vi "Encoder Quad Phase Detection.vi"(8 "Phase B":bool, 9 "Phase A":bool, 10 "Clear Error?":bool, 11 "Enable?":bool) -> (1 "Signal":bool, 2 "Backward?":bool, 3 "Error":bool)   [LabVIEW 2019]
uses:
  Encoder States.ctl
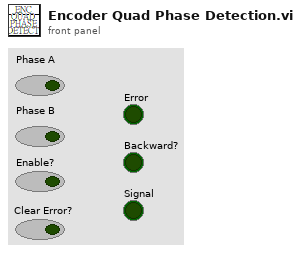
[diagram p1: front panel]
types:
  T1 = typedef "Encoder States.ctl" = fxp<+,3,3>
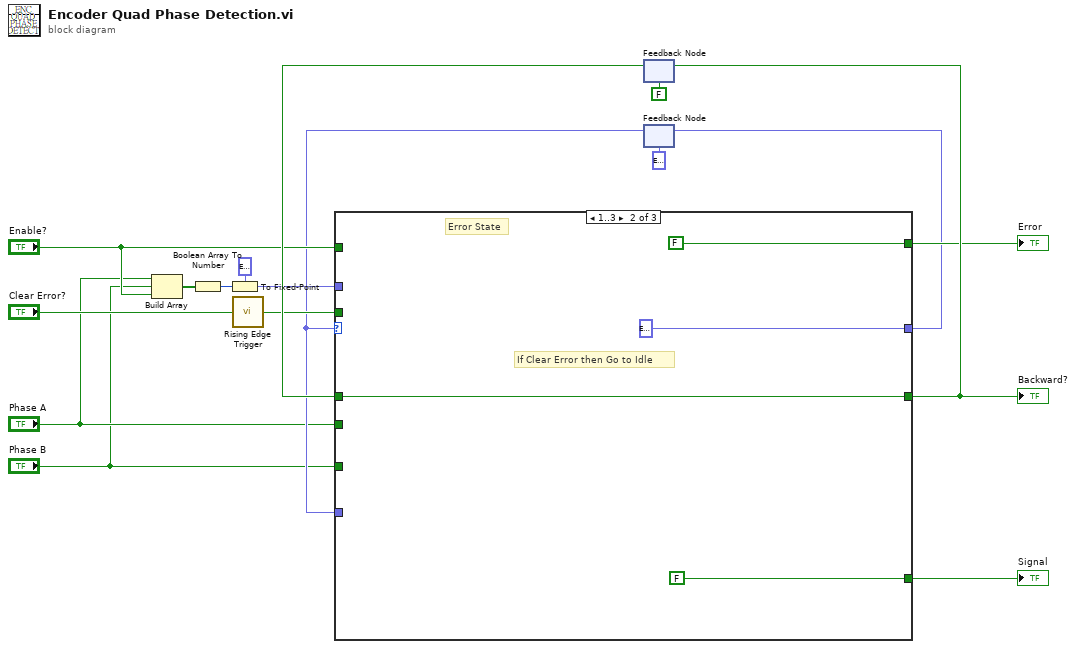
[diagram p0: block diagram]
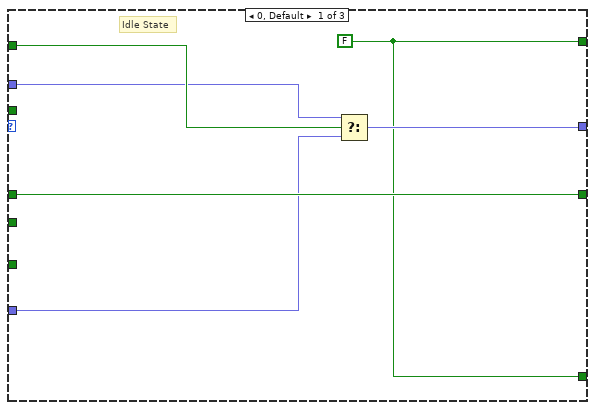
[diagram p2: hidden frame]
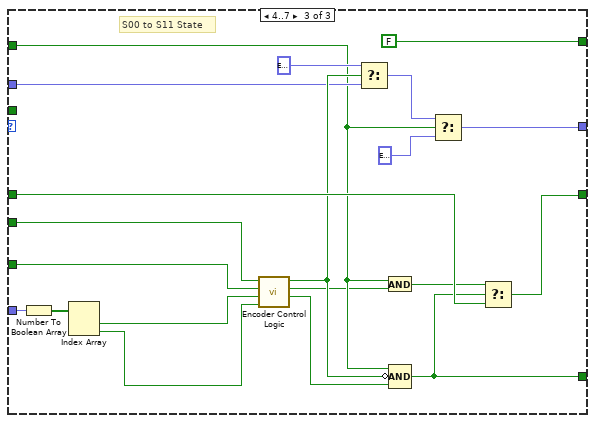
[diagram p3: hidden frame]
diagram:
  n1 = Build Array("Phase A", "Phase B", "Enable?") -> (w6:bool[])
  n2 = Boolean Array To Number(Boolean array=w6) -> (number=w5:u8)
  n3 = To Fixed-Point(fixed-point type=T1 0.0 ("Numeric"), number=w5) -> (fixed-point=w3:T1)
  n4 = call "Rising Edge Trigger.vi"("Signal"="Clear Error?") -> ("Trigger?"=w9:bool)
  n5 = feedback #1(FALSE ("Direction")) -> (w11:bool)
  n6 = feedback #2(T1 0.0) -> (w7:T1)
  n7 = case shown="1..3" w7 {
    tunnel: "Enable?" -> [w23 _ w34]
    tunnel: [w21 T1 0.0 ("t") w38] -> w13
    tunnel: [w19 FALSE ("Error") FALSE ("Error")] -> w15
    tunnel: w3 -> [w22 _ w42]
    tunnel: w11 -> [w20 w26 w47]
    tunnel: [w20 w26 w46] -> w16
    tunnel: [w19 FALSE ("Error") w36] -> w17
    tunnel: w9 -> [_ _ _]
    tunnel: "Phase B" -> [_ _ w44]
    tunnel: "Phase A" -> [_ _ w45]
    tunnel: w7 -> [w18 _ w29]
    frame 0, Default {
      w19 = FALSE ("Error")
      # "Idle State"
      n8 = Select(t=w22, s=w23, f=w18) -> (s? t:f=w21:T1)
    }
    frame 1..3 {
      # "Error State"
      # "If Clear Error then Go to Idle"
    }
    frame 4..7 {
      # "S00 to S11 State"
      n9 = Number To Boolean Array(number=w29) -> (Boolean array=w31:bool[])
      n10 = Index Array(array=w31) -> (element #1=w30:bool, element #2=w28:bool)  [unwired: 2 in]
      n11 = call "Encoder Control Logic.vi"("Prev Phase B (State Bit 1)"=w28, "Prev Phase A (State Bit 0)"=w30, "Phase B"=w44, "Phase A"=w45) -> ("Count?"=w33:bool, "Backward?"=w32:bool, "Error Occurred?"=w43:bool)  [unwired: 5 in]
      n12 = Select(t=T1 1.0, s=w43, f=w42) -> (s? t:f=w40:T1)
      n13 = And(x=w34, y=w32) -> (x .and. y?=w35:bool)
      n14 = Compound Arithmetic op=AND(w34, invert w43, w33) -> (w36:bool)
      n15 = Select(t=w40, s=w34, f=T1 0.0) -> (s? t:f=w38:T1)
      n16 = Select(t=w35, s=w36, f=w47) -> (s? t:f=w46:bool)
    }
  }
  "Backward?" <- w16
  "Signal" <- w17
  "Error" <- w15
  n17 = feedback-in #1(w16) -> ()
  n18 = feedback-in #2(w13) -> ()
